vi "C867_Connect.vi"(8 "error in":errorcluster caption="entrée d'erreur") -> (0 "error out":errorcluster caption="sortie d'erreur", 3 "ID":i32 caption="Numérique")   [LabVIEW 2026]
uses:
  Controls/TypeDef_FGV.ctl
  C867-VIs/Low Level/PI_GCS2_DLL_x64.dll
panel:
  in  "nBaudRate":i32=115200
  in  "nPortNr":i32=15
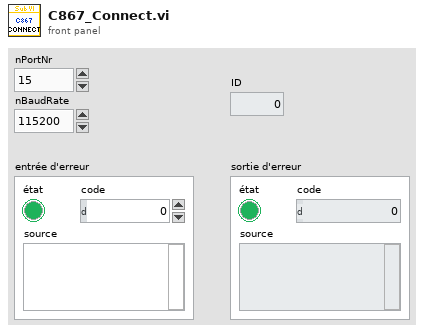
[diagram p1: front panel]
types:
  T1 = typedef "TypeDef_FGV.ctl" = enum16{"Initialize", "Write", "Read"}
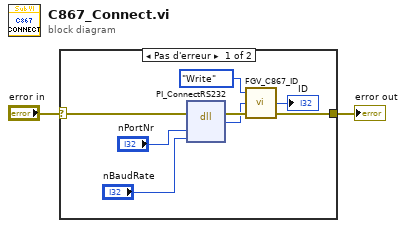
[diagram p0: block diagram]
diagram:
  n1 = case shown="Pas d'erreur" "error in" {
    selector: "error in" -> [w10 w11]
    tunnel: [w6 w11] -> w1
    frame No Error {
      n2 = dll-call lib="C:/Users/Sebastien/Documents/GitHub/LABVIEW-Useful-codes/Device_control/PC-C867-IO Control/v0.2/SubVI/PI-C867/C867-VIs/Low Level/PI_GCS2_DLL_x64.dll" fn="PI_ConnectRS232"(error in=w10, "nPortNr"="nPortNr", "nBaudRate"="nBaudRate") -> (error out=w4:errorcluster, "ID"=w3:i32)  [unwired: 4 in, 1 out]
      n3 = call "FGV_C867_ID.vi"("error in"=w4, "ID"=w3, "Action"=TypeDef_FGV."Write") -> ("error out"=w6:errorcluster, "ID"=→"ID":i32)  [unwired: 1 in]
    }
    frame Error {
    }
  }
  "error out" <- w1
